vi "File.Copy with Overwrite.vi"(8 "error in (no error)":errorcluster, 9 "Dest is Dir(F)/File(T)":bool, 10 "Destination":path, 11 "Source":path) -> (0 "error out":errorcluster, 2 "Files Copied":i32, 3 "Destination Dup":path)   [LabVIEW 2024, in "EQMF.lvlib" / "File Utils.lvlib"]
uses:
  File Utils.lvlib
panel:
  out "Cmd":string
  out "RtnCode":i32
  out "StdErr":string
  out "StdOut":string
  # "If Source is Dir then Dest must be Dir\nFiles and subfolders are copied from the source path to the destination path.\nNOTE: In order to copy a folder from a source location to a destination location, the source and destination path must include the folder."
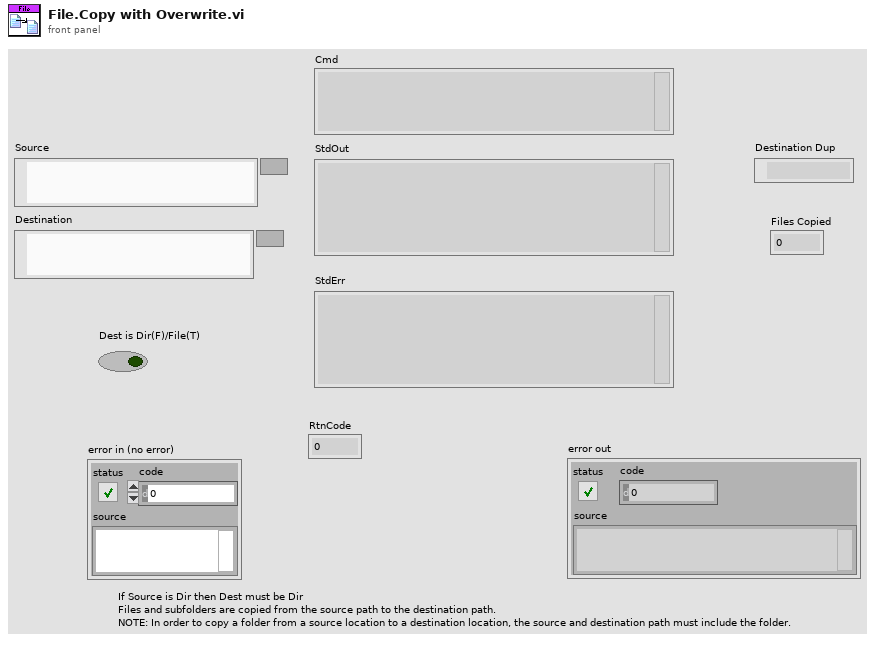
[diagram p1: front panel]
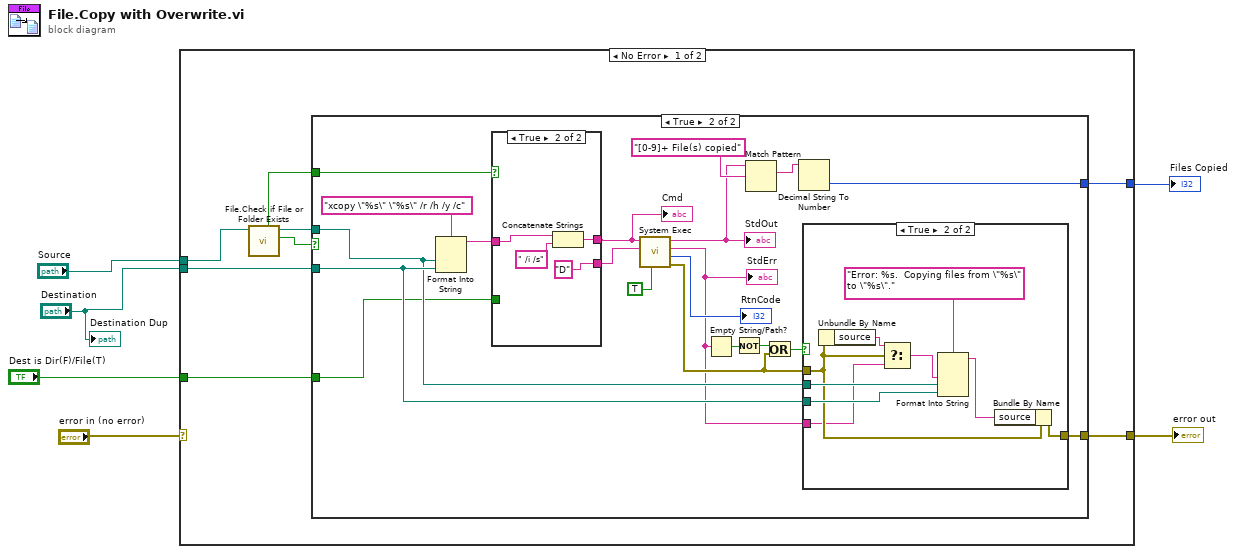
[diagram p0: block diagram]
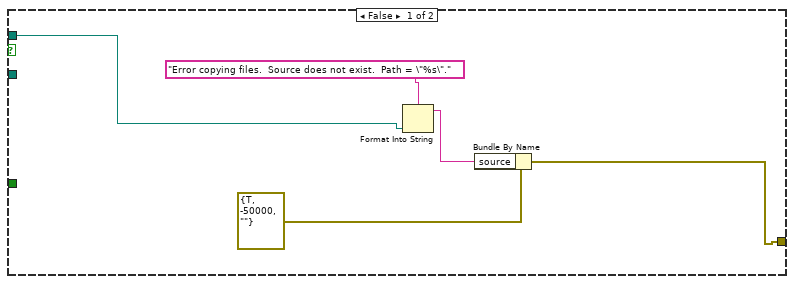
[diagram p2: hidden frame]
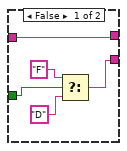
[diagram p3: hidden frame]
diagram:
  n1 = case shown="No Error" "error in (no error)" {
    selector: "error in (no error)" -> [_ w58]
    tunnel: "Source" -> [w11 _]
    tunnel: [w12 w58] -> w5
    tunnel: "Destination" -> [w13 _]
    tunnel: [w14 _] -> w2
    tunnel: "Dest is Dir(F)/File(T)" -> [w7 _]
    frame No Error {
      n2 = call "File.Check if File or Folder Exists.vi"("Path"=w11) -> ("Exists"=w9:bool, "Dup Path"=w10:path, "IsDir"=w8:bool)  [unwired: 6 in, 2 out]
      n3 = case shown="True" w9 {
        tunnel: [_ w33] -> w14
        tunnel: w13 -> [_ w32]
        tunnel: [w16 w31] -> w12
        tunnel: w10 -> [w17 w30]
        tunnel: w8 -> [_ w28]
        tunnel: w7 -> [_ w25]
        frame False {
          n4 = Format Into String(format string="Error copying files.  Source does not exist.  Path = \"%s\".", w17) -> (resulting string=w18:string)  [unwired: 2 in, 1 out]
          n5 = Bundle By Name(cluster=errorcluster {"status"=TRUE, "code"=-50000, "source"=""} ("error constant"), "source"=w18) -> (w16:errorcluster)
        }
        frame True {
          n6 = Format Into String(format string="xcopy \"%s\" \"%s\" /r /h /y /c", w30, w32) -> (resulting string=w29:string)  [unwired: 2 in, 1 out]
          n7 = case shown="True" w28 {
            tunnel: w29 -> [w44 w46]
            tunnel: [w44 w48] -> w27
            tunnel: [w40 "D" ("standard input")] -> w26
            tunnel: w25 -> [w41 _]
            frame False {
              n8 = Select(t="F" ("standard input"), s=w41, f="D" ("standard input")) -> (s? t:f=w40:string)
            }
            frame True {
              n9 = Concatenate Strings(w46, " /i /s") -> (w48:string)
            }
          }
          "Cmd" <- w27
          n10 = call <vilib>:"System Exec.vi"("run minimized? (F)"=TRUE, "standard input"=w26, "command line"=w27) -> ("error out"=w21:errorcluster, "return code"=→"RtnCode":i32, "standard error"=w20:string, "standard output"=w35:string)  [unwired: 5 in]
          "StdErr" <- w20
          "StdOut" <- w35
          n11 = Empty String/Path?(string/path=w20) -> (empty?=w24:bool)
          n12 = Not(x=w24) -> (.not. x?=w23:bool)
          n13 = Match Pattern(string=w35, regular expression="[0-9]+ File(s) copied") -> (match substring=w34:string)  [unwired: 1 in, 3 out]
          n14 = Or(x=w23, y=w21) -> (x .or. y?=w22:bool)
          n15 = Decimal String To Number(string=w34) -> (number=w33:i32)  [unwired: 2 in, 1 out]
          n16 = case shown="True" w22 {
            tunnel: w30 -> [_ w55]
            tunnel: [_ w57] -> w31
            tunnel: w32 -> [_ w54]
            tunnel: w21 -> [_ w52]
            tunnel: w20 -> [_ w50]
            frame False {
            }
            frame True {
              n17 = Unbundle By Name(w52) -> ("source"=w51:string)
              n18 = Select(t=w51, s=w52, f=w50) -> (s? t:f=w49:string)
              n19 = Format Into String(format string="Error: %s.  Copying files from \"%s\" to \"%s\".", w49, w55, w54) -> (resulting string=w53:string)  [unwired: 2 in, 1 out]
              n20 = Bundle By Name(cluster=w52, "source"=w53) -> (w57:errorcluster)
            }
          }
        }
      }
    }
    frame Error {
    }
  }
  "error out" <- w5
  "Files Copied" <- w2
  "Destination Dup" <- "Destination"
